vi "HT-3015-Lutron-MRC-Humidity_Temperature_Logger.vi"(8 "error in (no error)":errorcluster) -> (0 "error out":errorcluster={"status"=TRUE, "code"=-1073807338, "source"="VISA Close in O3 ThermoScientific 49.vi"})   [LabVIEW 2013]
doc: "Use this template to build a VI to use as a subVI."
uses:
  <vilib>/Instr/_visa.llb/VISA Configure Serial Port (Instr).vi
  <vilib>/Utility/file.llb/Write To Spreadsheet File (string).vi
panel:
  out "Humidity and Temp(deg":cluster{dbl, dbl}
  out "RH or Temp?":string
  out "Polarity":string
  out "Decimal Point":string
  out "Reading":string
  in  "Emulation":bool
  in  "Serial Port Number":refnum<visa-resource-name>="COM3"
  in  "Save to File":bool=TRUE
  in  "file path":path=path "C:/Users/DMA2011/Desktop/o3Conc.txt"
  out "read buffer":string="o3 3353E-2 ppb\r"
  in  "stop":bool
  out "Waveform Chart":waveform(dbl)[](graph)
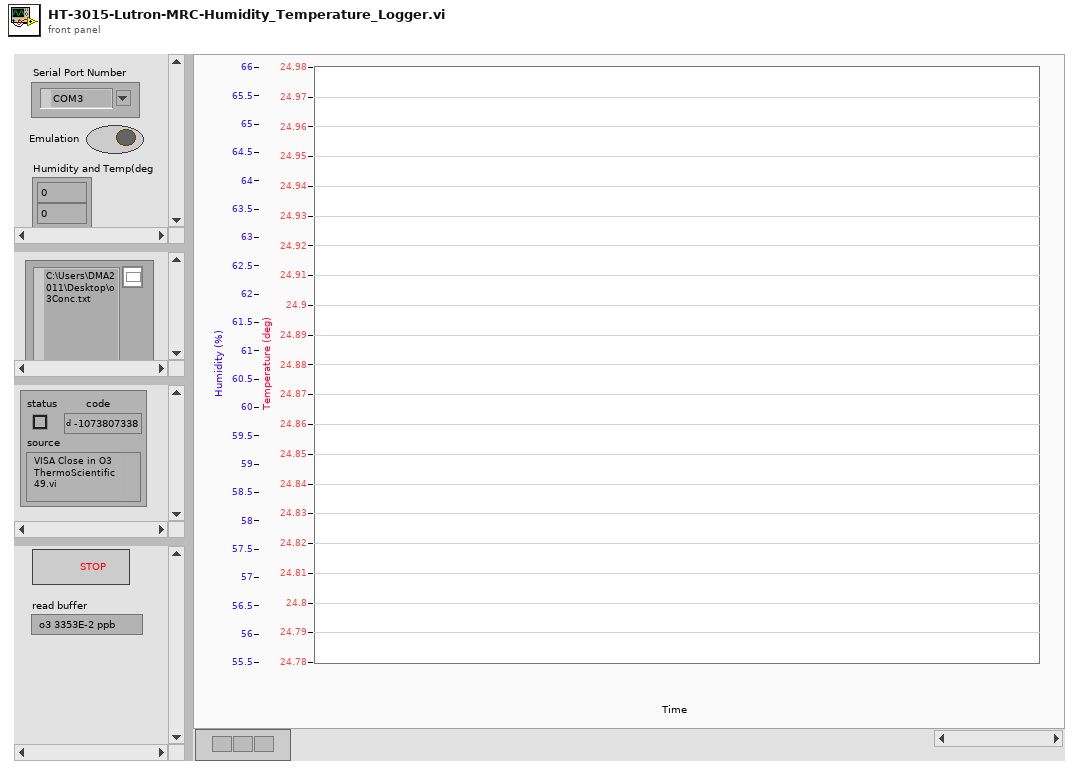
[diagram p1: front panel]
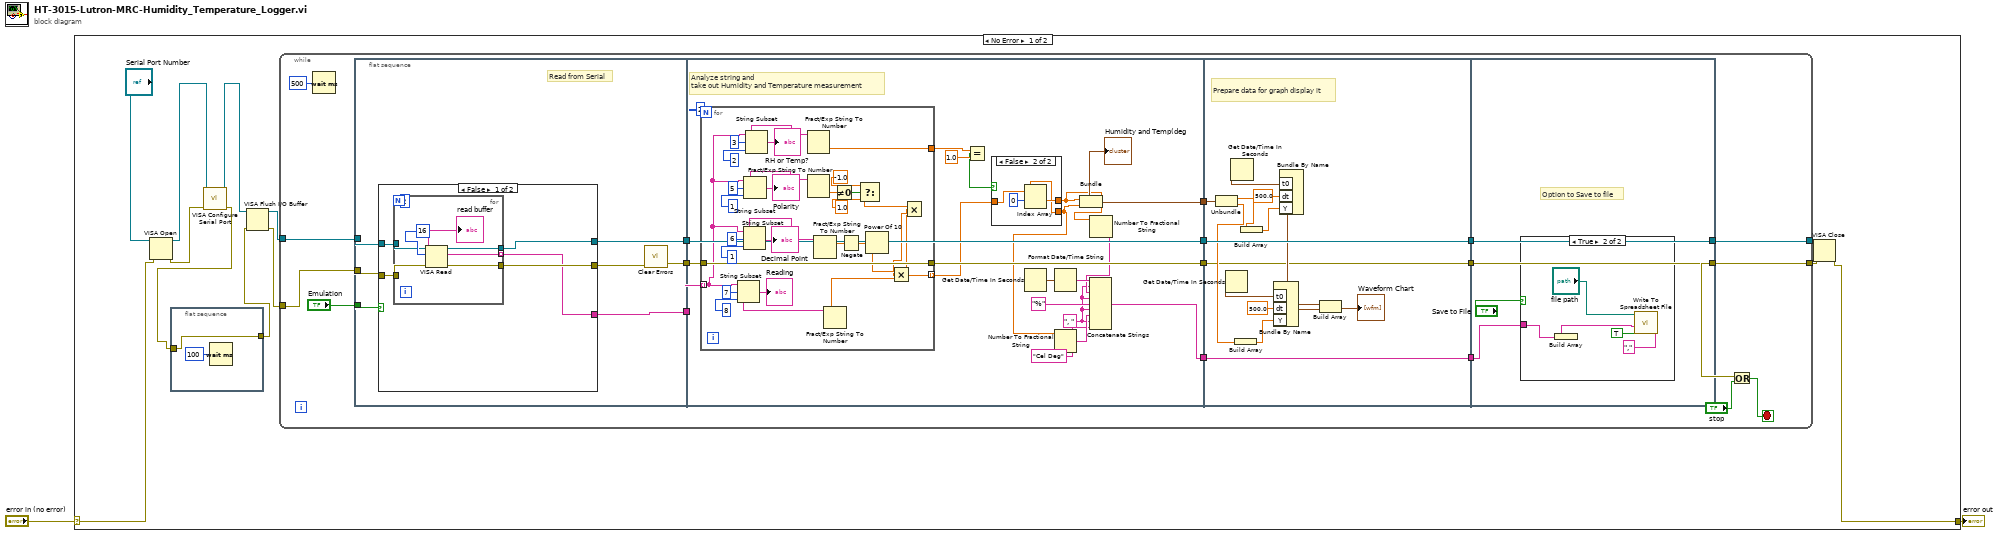
[diagram p0: block diagram]
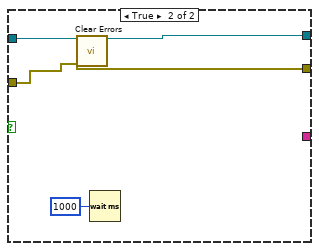
[diagram p2: hidden frame]
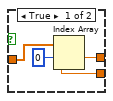
[diagram p3: hidden frame]
diagram:
  n1 = case shown="No Error" "error in (no error)" {
    selector: "error in (no error)" -> [w13 w136]
    tunnel: [w10 w136] -> w1
    frame No Error {
      n2 = VISA Open(error in (no error)=w13, VISA resource name="Serial Port Number") -> (VISA resource name=w9:refnum<visa-resource-name>, error out=w8:errorcluster)  [unwired: 3 in]
      n3 = flat-sequence {
        tunnel: w7 -> [w15]
        tunnel: [w15] -> w4
        frame #0 {
          n4 = Wait (ms)(milliseconds to wait=u32 100) -> ()  [unwired: 1 out]
        }
      }
      n5 = call-poly "VISA Configure Serial Port"("VISA resource name"=w9, "error in (no error)"=w8) -> ("VISA resource name out"=w6:refnum<visa-resource-name>, "error out"=w7:errorcluster)  [unwired: 12 in]
      n6 = VISA Flush I/O Buffer(VISA resource name=w6, error in (no error)=w4) -> (VISA resource name out=w5:refnum<visa-resource-name>, error out=w3:errorcluster)  [unwired: 1 in]
      n7 = while {
        tunnel: w5 -> [w34]
        tunnel: w3 -> [w28]
        tunnel: [w31] -> w12
        tunnel: [w33] -> w11
        stop <- w30 stop-if-true
        n8 = Wait (ms)(milliseconds to wait=u32 500) -> ()  [unwired: 1 out]
        n9 = flat-sequence {
          tunnel: w34 -> [w41]
          tunnel: "Emulation" -> [w39]
          tunnel: w28 -> [w37]
          tunnel: [w40] -> w27
          tunnel: [w35] -> w26
          tunnel: [w38] -> w25
          tunnel: w27 -> [w77]
          tunnel: w26 -> [w74]
          tunnel: w25 -> [w73]
          tunnel: [w77] -> w24
          tunnel: [w72] -> w21
          tunnel: [w75] -> w19
          tunnel: [w65] -> w17
          tunnel: w24 -> [w126]
          tunnel: [w126] -> w23
          tunnel: [w113] -> w22
          tunnel: w21 -> [w113]
          tunnel: [w123] -> w20
          tunnel: w19 -> [w123]
          tunnel: w17 -> [w118]
          tunnel: [w129] -> w31
          tunnel: [w130] -> w33
          tunnel: w23 -> [w130]
          tunnel: w22 -> [w129]
          tunnel: w20 -> [w127]
          frame #0 {
            # "Read from Serial"
            n10 = case shown="False" w39 {
              tunnel: w41 -> [w44 w57]
              tunnel: [w46 w57] -> w40
              tunnel: [w45 _] -> w38
              tunnel: [w47 w54] -> w36
              tunnel: w37 -> [w43 w55]
              frame False {
                n11 = for {
                  N: 2 -> [_]
                  tunnel: [w52] -> w47
                  tunnel: [w51] -> w46
                  tunnel: [w50] -> w45 mode=indexing
                  tunnel: w44 -> [w49]
                  tunnel: w43 -> [w48]
                  n12 = VISA Read(VISA resource name=w49, byte count=u32 16, error in (no error)=w48) -> (VISA resource name out=w51:refnum<visa-resource-name>, read buffer=w50:string, error out=w52:errorcluster)  [unwired: 1 out]
                  "read buffer" <- w50
                }
              }
              frame True {
                n13 = call <vilib>:"Clear Errors.vi"("error in (no error)"=w55) -> ("error out"=w54:errorcluster)  [unwired: 6 in]
                n14 = Wait (ms)(milliseconds to wait=u32 1000) -> ()  [unwired: 1 out]
              }
            }
            n15 = call <vilib>:"Clear Errors.vi"("error in (no error)"=w36) -> ("error out"=w35:errorcluster)  [unwired: 6 in]
          }
          frame #1 {
            w59 = ", " ("string")
            # "Analyze string and\ntake out Humidity and Temperature measurement"
            n16 = for {
              N: 2 -> [_]
              tunnel: w74 -> [w109]
              tunnel: w73 -> [w88] mode=indexing
              tunnel: [w109] -> w72
              tunnel: [w91] -> w67 mode=indexing
              tunnel: [w86] -> w69
              n17 = String Subset(string=w88, offset (0)=7, length (rest)=8 ("length (rest)")) -> (substring=w106:string)
              "Reading" <- w106
              n18 = String Subset(string=w88, offset (0)=6, length (rest)=1 ("length (rest)")) -> (substring=w105:string)
              "Decimal Point" <- w105
              n19 = String Subset(string=w88, offset (0)=5, length (rest)=1 ("length (rest)")) -> (substring=w98:string)
              "Polarity" <- w98
              n20 = String Subset(string=w88, offset (0)=3, length (rest)=2 ("length (rest)")) -> (substring=w87:string)
              "RH or Temp?" <- w87
              n21 = Fract/Exp String To Number(string=w87) -> (number=w86:dbl)  [unwired: 3 in, 1 out]
              n22 = Fract/Exp String To Number(string=w98) -> (number=w97:dbl)  [unwired: 3 in, 1 out]
              n23 = Fract/Exp String To Number(string=w105) -> (number=w104:dbl)  [unwired: 3 in, 1 out]
              n24 = Fract/Exp String To Number(string=w106) -> (number=w101:dbl)  [unwired: 3 in, 1 out]
              n25 = Not Equal To 0?(x=w97) -> (x != 0?=w96:bool)
              n26 = Negate(x=w104) -> (-x=w103:dbl)
              n27 = Select(t=-1.0, s=w96, f=1.0) -> (s? t:f=w93:dbl)
              n28 = Power Of 10(x=w103) -> (10^x=w102:dbl)
              n29 = Multiply(x=w102, y=w101) -> (x*y=w92:dbl)
              n30 = Multiply(x=w93, y=w92) -> (x*y=w91:dbl)
            }
            n31 = Equal?(x=w69, y=1.0) -> (x = y?=w66:bool)
            n32 = case shown="False" w66 {
              tunnel: w67 -> [w81 w85]
              tunnel: [w79 w83] -> w64
              tunnel: [w78 w82] -> w61
              frame True {
                n33 = Index Array(array=w81, index #1=0 ("index")) -> (element #1=w79:dbl, element #2=w78:dbl)  [unwired: 1 in]
              }
              frame False {
                n34 = Index Array(array=w85, index #1=0 ("index")) -> (element #1=w82:dbl, element #2=w83:dbl)  [unwired: 1 in]
              }
            }
            n35 = Get Date/Time In Seconds() -> (seconds since 1Jan1904=w76:timestamp)
            n36 = Format Date/Time String(seconds (now)=w76) -> (date/time string=w71:string)  [unwired: 2 in]
            n37 = Number To Fractional String(number=w61) -> (F-format string=w60:string)  [unwired: 3 in]
            n38 = Bundle(w64, w61) -> (w65:cluster{dbl, dbl})  [unwired: 1 in]
            "Humidity and Temp(deg" <- w65
            n39 = Number To Fractional String(number=w64) -> (F-format string=w63:string)  [unwired: 3 in]
            n40 = Concatenate Strings(w71, w59, w63, w59, "%" ("string"), w59, w60, w59, "Cel Deg" ("string")) -> (w75:string)
          }
          frame #2 {
            # "Prepare data for graph display it"
            n41 = Unbundle(w118) -> (w117:dbl, w116:dbl)
            n42 = Get Date/Time In Seconds() -> (seconds since 1Jan1904=w125:timestamp)
            n43 = Get Date/Time In Seconds() -> (seconds since 1Jan1904=w119:timestamp)
            n44 = Build Array(w116) -> (w122:dbl[])
            n45 = Build Array(w117) -> (w121:dbl[])
            n46 = Bundle By Name("t0"=w125, "dt"=500.0, "Y"=w122) -> (w115:waveform(dbl))  [unwired: 1 in]
            n47 = Bundle By Name("t0"=w119, "dt"=500.0, "Y"=w121) -> (w114:waveform(dbl))  [unwired: 1 in]
            n48 = Build Array(w114, w115) -> (→"Waveform Chart":waveform(dbl)[])
          }
          frame #3 {
            # "Option to Save to file"
            n49 = case shown="True" "Save to File" {
              tunnel: w127 -> [_ w132]
              frame False {
              }
              frame True {
                n50 = Build Array(w132) -> (w131:string[])
                n51 = call-poly <vilib>:"Write To Spreadsheet File.vi"("delimiter (\\t)"="," ("delimiter (\\t)"), "append to file? (new file:F)"=TRUE, "1D data"=w131, "file path (dialog if empty)"="file path") -> ()  [unwired: 4 in, 1 out]
              }
            }
          }
        }
        n52 = Or(x=w31, y="stop") -> (x .or. y?=w30:bool)
      }
      n53 = VISA Close(VISA resource name=w11, error in (no error)=w12) -> (error out=w10:errorcluster)
    }
    frame Error {
    }
  }
  "error out" <- w1
